vi "Create MetaData Channel_ex.vi"() -> ()   [LabVIEW 2019]
uses:
  <vilib>/NI VeriStand/Custom Device API/Custom Device Item Ref.ctl
  Control 11.ctl
  Control 13.ctl
  Control 12.ctl
  Scripting API/Polymorphic/Create Channel/Create Command Array Channel_Type Cast.vi
  Scripting API/Scripting API.lvlib
  <vilib>/NI VeriStand/Custom Device API/Custom Device API.lvlib
panel:
  out "Message Refnum Out":T1=18446744073709551615 format="%.0x"
  out "Channel Refnums":T1[](array[typedef]) format="%.0x"
  out "Error Out":errorcluster
  in  "Message Refnum In":T1=18446744073709551615 format="%.0x"
  in  "Error In":errorcluster
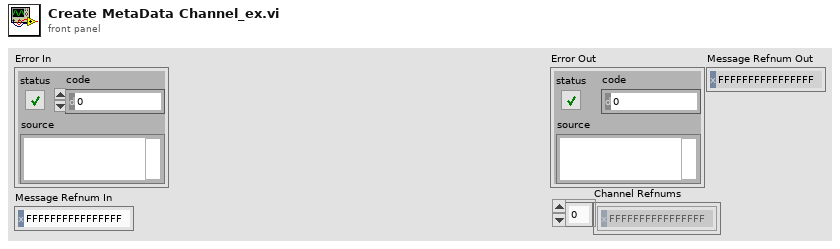
[diagram p1: front panel]
types:
  T1 = typedef "Custom Device API.lvlib/Custom Device Item Ref.ctl" = u64
  T2 = typedef "Control 11.ctl" = cluster{"Elements":cluster{"Default Value":dbl, "Units":string}[], "Delimiter":string, "Type":T3, "Endian":T4}
  T3 = typedef "Control 13.ctl" = enum16{"DBL"}
  T4 = typedef "Control 12.ctl" = enum16{"Big", "Little", "Native"}
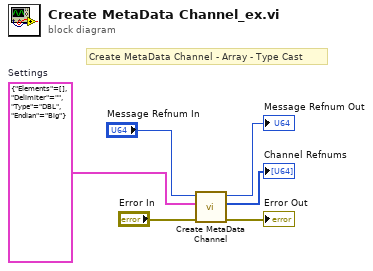
[diagram p0: block diagram]
diagram:
  w5 = T2 {"Elements"=[], "Delimiter"="", "Type"=enum."DBL", "Endian"=enum."Big"}  # Settings
  # "Create MetaData Channel - Array - Type Cast"
  n1 = call-poly "Create MetaData Channel.vi"("Error In"="Error In", "Settings"=w5, "Message Refnum In"="Message Refnum In") -> ("Error Out"=→"Error Out":errorcluster, "Channel Refnums"=→"Channel Refnums":T1[], "Message Refnum Out"=→"Message Refnum Out":T1)  [unwired: 6 in]
